vi "Drive Published Globals.vi"() -> ()   [LabVIEW 2016]
doc: "This is used primarily to publish values that other subsystems or user code may want to read periodically. It may also contain some settings such as debug switches or implementation selections that are independent of the operating mode of the subsystem."
panel:
  in  "Start angle":dbl
  in  "Initial Offset":dbl
  in  "pigeon":dbl
  in  "score":dbl=nan
  in  "Gear Rect":T1={"Left"=nan, "Top"=nan, "Right"=nan, "Bottom"=nan}
  in  "Encoder Right":dbl
  in  "Encoder Left":dbl
  # "Tip: The global is a good way publish state or\ninformational/debugging values.\nIt is not  advised that you put setpoint values here."
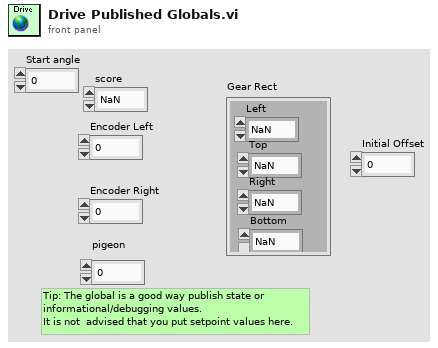
[diagram p1: front panel]
types:
  T1 = cluster{"Left":dbl, "Top":dbl, "Right":dbl, "Bottom":dbl}
diagram:
